vi "Find Matching Nets.vi"(9 "Amount Processed":refnum<vi>, 10 "Progress Reference":refnum<vi>, 11 "Refnums 1":refnum<vi>[](array[refnum])) -> (2 "Nets Found":T5(array[cluster]), 3 "VIs matching Criteria":T1[](array[typedef]))   [LabVIEW 2019]
uses:
  Advanced Search.llb/Terminal Filter Output.ctl
  Advanced Search.llb/Terminals within Selection and GObject.ctl
  Advanced Search.llb/Project Items.ctl
  Advanced Search.llb/Control 2.ctl
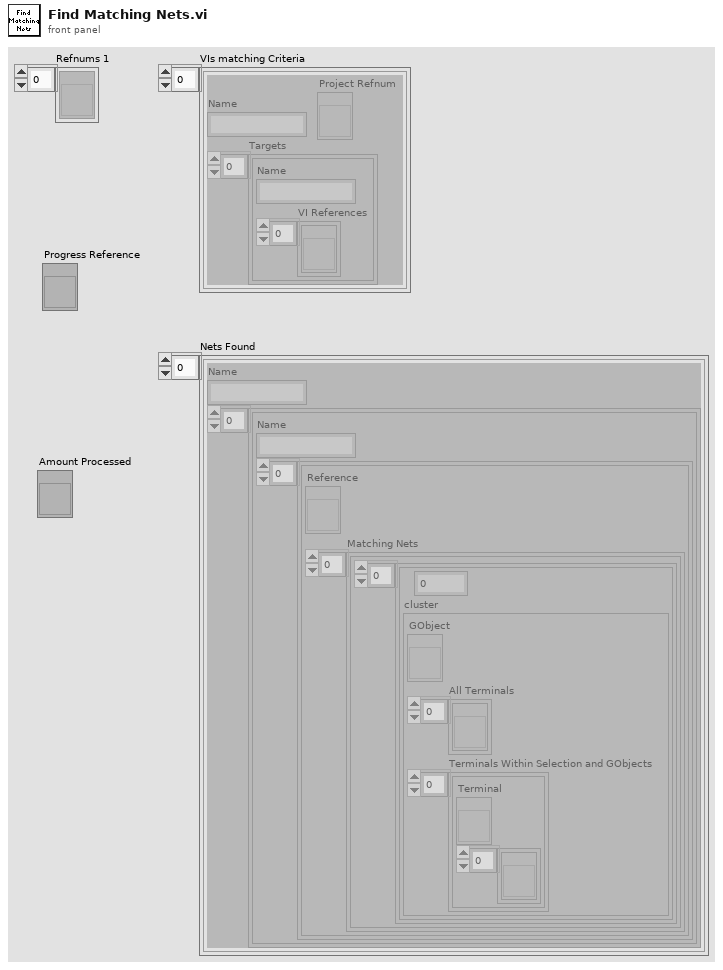
[diagram p1: front panel]
types:
  T1 = typedef "Project Items.ctl" = cluster{"Name":string, "Targets":T2[], "Project Refnum":refnum<vi>}
  T2 = typedef "Control 2.ctl" = cluster{"Name":string, "VI References":refnum<vi>[]}
  T3 = typedef "Terminal Filter Output.ctl" = cluster{"GObject":refnum<vi>, "All Terminals":refnum<vi>[], "Terminals Within Selection and GObjects":T4[]}
  T4 = typedef "Terminals within Selection and GObject.ctl" = cluster{"Terminal":refnum<vi>, "Attached GObjects":refnum<vi>[]}
  T5 = cluster{"Name":string, cluster{"Name":string, cluster{"Reference":refnum<vi>, "Matching Nets":cluster{cluster{i32, "cluster":T3}[]}[]}[]}[]}[]
  T6 = typedef "Filtered VI.ctl" = cluster{"Reference":refnum<vi>, "AllObjs[]":refnum<vi>[]}
  T7 = cluster{"Reference":refnum<vi>, "Matching Nets":cluster{cluster{i32, "cluster":T3}[]}[]}
  T8 = cluster{"Name":string, cluster{"Reference":refnum<vi>, "Matching Nets":cluster{cluster{i32, "cluster":T3}[]}[]}[]}
  T9 = cluster{"Name":string, cluster{"Name":string, cluster{"Reference":refnum<vi>, "Matching Nets":cluster{cluster{i32, "cluster":T3}[]}[]}[]}[]}
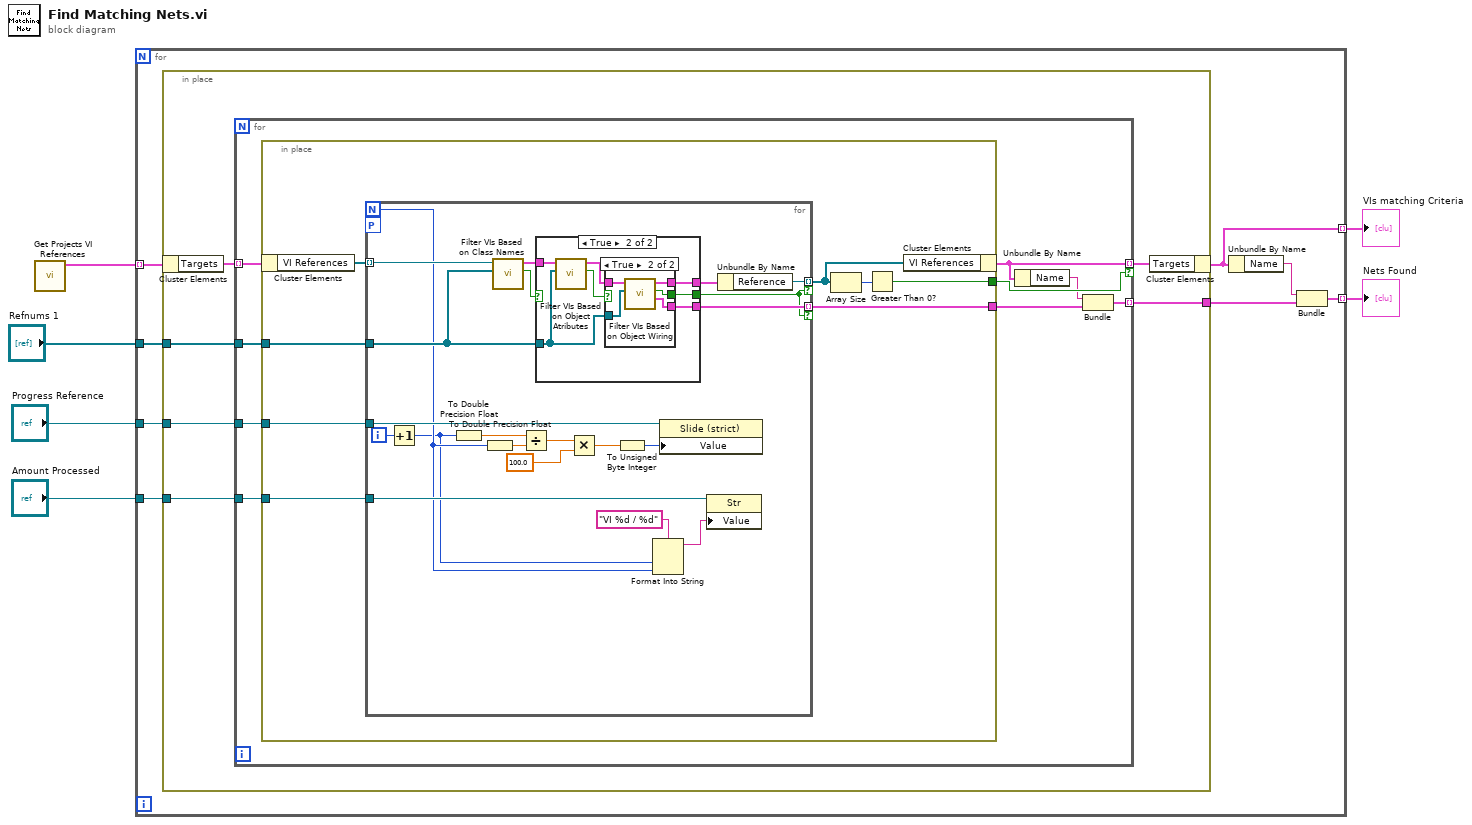
[diagram p0: block diagram]
diagram:
  n1 = call "Get Projects VI References.vi"() -> ("Project Items"=w4:T1[])  [unwired: 10 in, 1 out]
  n2 = for {
    tunnel: "Refnums 1" -> [w14]
    tunnel: w4 -> [w13] mode=indexing
    tunnel: [w12] -> w5 mode=indexing
    tunnel: [w9] -> w6 mode=indexing
    tunnel: "Progress Reference" -> [w8]
    tunnel: "Amount Processed" -> [w7]
    n3 = in-place {
      in-place-border: w14 -> [w20]
      in-place-border: [w17] -> w10
      in-place-border: w8 -> [w16]
      in-place-border: w7 -> [w15]
      n4 = in-place-cluster #1(w13) -> ("Targets"=w19:T2[])
      n5 = for {
        tunnel: w20 -> [w29]
        tunnel: w19 -> [w28] mode=indexing
        tunnel: [w23] -> w18 mode=indexing if=w27
        tunnel: [w25] -> w17 mode=indexing
        tunnel: w16 -> [w22]
        tunnel: w15 -> [w21]
        n6 = in-place {
          in-place-border: w29 -> [w34]
          in-place-border: [w35] -> w27
          in-place-border: [w33] -> w24
          in-place-border: w22 -> [w31]
          in-place-border: w21 -> [w30]
          n7 = in-place-cluster #2(w28) -> ("VI References"=w37:refnum<vi>[])
          n8 = for {
            N -> [w42]
            tunnel: w37 -> [w58] mode=indexing
            tunnel: w34 -> [w56]
            tunnel: [w55] -> w33 mode=indexing if=w51
            tunnel: [w53] -> w32 mode=indexing if=w51
            tunnel: w31 -> [w48]
            tunnel: w30 -> [w46]
            workers-P: _ -> [_]
            i -> [w43]
            n9 = Increment(x=w43) -> (x+1=w41:i32)
            n10 = To Double Precision Float(number=w41) -> (double precision float=w38:dbl)
            n11 = To Double Precision Float(number=w42) -> (double precision float=w39:dbl)
            n12 = call "Filter VIs Based on Class Names.vi"("Selected GObject References"=w56, "VI Reference"=w58) -> ("Valid VI"=w52:bool, "Filtered VI"=w57:T6)  [unwired: 7 in, 1 out]
            n13 = Divide(x=w38, y=w39) -> (x/y=w50:dbl)
            n14 = case shown="True" w52 {
              tunnel: w57 -> [_ w65]
              tunnel: w56 -> [_ w63]
              tunnel: [_ w62] -> w55
              tunnel: [_ w61] -> w54
              tunnel: [_ w59] -> w51
              frame False {
              }
              frame True {
                n15 = call "Filter VIs Based on Object Atributes.vi"("Selected GObject References"=w63, "Filtered VI In"=w65) -> ("Valid VI"=w60:bool, "Filtered VI Out"=w64:T6)  [unwired: 8 in]
                n16 = case shown="True" w60 {
                  tunnel: w64 -> [_ w70]
                  tunnel: w63 -> [_ w69]
                  tunnel: [_ w68] -> w62
                  tunnel: [_ w67] -> w61
                  tunnel: [_ w66] -> w59
                  frame False {
                  }
                  frame True {
                    n17 = call "Filter VIs Based on Object Wiring.vi"("Selected Refnums"=w69, "Filtered VI In"=w70) -> ("Found Nets"=w68:T7, "Valid VI"=w66:bool, "Filtered VI Out"=w67:T6)  [unwired: 7 in]
                  }
                }
              }
            }
            n18 = Multiply(x=w50, y=100.0) -> (x*y=w47:dbl)
            n19 = To Unsigned Byte Integer(number=w47) -> (unsigned 8bit integer=w40:u8)
            n20 = Format Into String(format string="VI %d / %d", w41, w42) -> (resulting string=w44:string)  [unwired: 2 in, 1 out]
            n21 = property class="Slide (strict)"(reference=w48, "Value"=w40) -> ()  [unwired: 1 in, 2 out]
            n22 = property class="Str"(reference=w46, "Value"=w44) -> ()  [unwired: 1 in, 2 out]
            n23 = Unbundle By Name(w54) -> ("Reference"=w53:refnum<vi>)
          }
          n24 = Array Size(array=w32) -> (size(s)=w36:i32)
          n25 = Greater Than 0?(x=w36) -> (x > 0?=w35:bool)
          n26 = in-place-cluster #2("VI References"=w32) -> (w23:T2)
        }
        n27 = Unbundle By Name(w23) -> ("Name"=w26:string)
        n28 = Bundle("Name"=w26, w24) -> (w25:T8)  [unwired: 1 in]
      }
      n29 = in-place-cluster #1("Targets"=w18) -> (w12:T1)
    }
    n30 = Unbundle By Name(w12) -> ("Name"=w11:string)
    n31 = Bundle("Name"=w11, w10) -> (w9:T9)  [unwired: 1 in]
  }
  "Nets Found" <- w6
  "VIs matching Criteria" <- w5
